vi "Exit Loop.vi"(0 "Diagram in":refnum<vi>, 1 "Loop Terminal Types":T1[](array[typedef]), 5 "Outputs":refnum<vi>[](array[refnum]), 7 "Shift Registers":refnum<vi>[](array[refnum]), 9 "Conditional Terminals":refnum<vi>[](array[refnum]), 11 "error in (no error)":errorcluster) -> (4 "Diagram out":refnum<vi>, 6 "Outputs":refnum<vi>[](array[refnum]), 8 "Shift Registers":refnum<vi>[](array[refnum]), 15 "error out":errorcluster)   [LabVIEW 2015, in "Scripting.lvlib"]
uses:
  Scripting.lvlib
  Loop Terminal Type.ctl
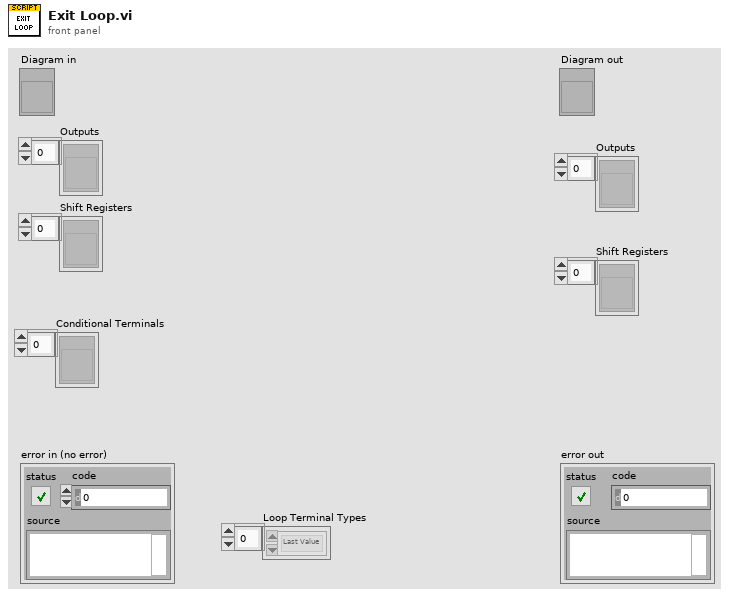
[diagram p1: front panel]
types:
  T1 = typedef "Scripting.lvlib/Loop Terminal Type.ctl" = enum16{"Last Value", "Indexing", "Concatenating"}
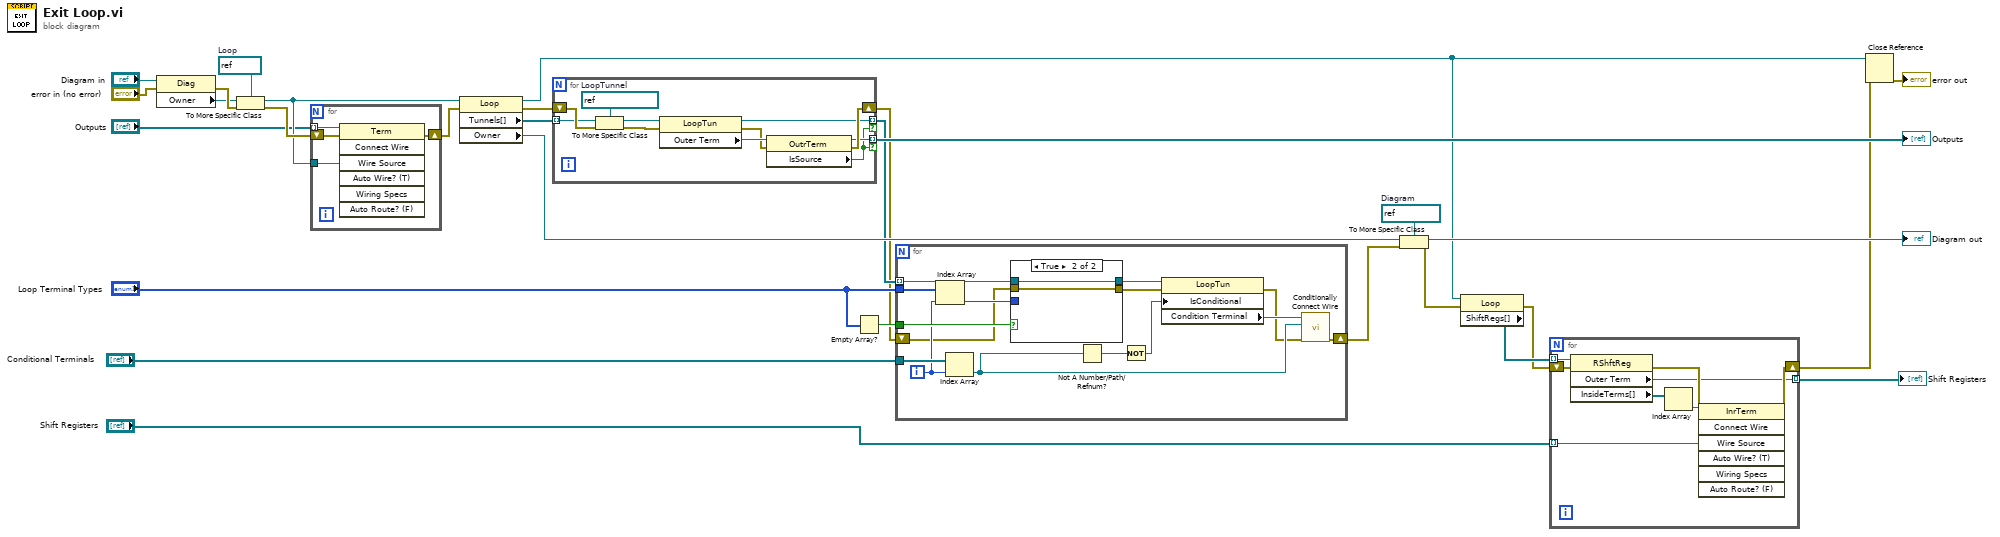
[diagram p0: block diagram]
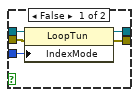
[diagram p2: hidden frame]
diagram:
  w25 = refnum<vi> refnum  # Diagram
  w27 = refnum<vi> refnum  # Loop
  n1 = property class="Diag"(reference="Diagram in", error in="error in (no error)") -> (error out=w28:errorcluster, "Owner"=w26:refnum<vi>)  [unwired: 1 out]
  n2 = To More Specific Class(target class=w27, reference=w26, error in=w28) -> (specific class reference=w24:refnum<vi>, error out=w29:errorcluster)
  n3 = for {
    tunnel: w24 -> [w32]
    shift-right: [w31] -> w23
    shift-left: w29 -> [w33]
    tunnel: "Outputs" -> [w30] mode=indexing
    n4 = invoke class="Term" method="Connect Wire"(reference=w30, error in=w33, "Wire Source"=w32) -> (error out=w31:errorcluster)  [unwired: 4 in, 6 out]
  }
  n5 = property class="Loop"(reference=w24, error in=w23) -> (reference out=w11:refnum<vi>, error out=w14:errorcluster, "Tunnels[]"=w15:refnum<vi>[], "Owner"=w16:refnum<vi>)
  n6 = for {
    tunnel: w15 -> [w38] mode=indexing
    tunnel: [w40] -> w18 mode=indexing if=w34
    shift-right: [w41] -> w3
    shift-left: w14 -> [w44]
    tunnel: [w35] -> w7 mode=indexing if=w34
    w36 = refnum<vi> refnum  # LoopTunnel
    n7 = To More Specific Class(target class=w36, reference=w38, error in=w44) -> (specific class reference=w37:refnum<vi>, error out=w39:errorcluster)
    n8 = property class="LoopTun"(reference=w37, error in=w39) -> (reference out=w35:refnum<vi>, error out=w42:errorcluster, "Outer Term"=w43:refnum<vi>)
    n9 = property class="OutrTerm"(reference=w43, error in=w42) -> (reference out=w40:refnum<vi>, error out=w41:errorcluster, "IsSource"=w34:bool)
  }
  "Outputs" <- w18
  n10 = Empty Array?(array="Loop Terminal Types") -> (empty?=w5:bool)
  n11 = for {
    tunnel: w7 -> [w59] mode=indexing
    tunnel: "Loop Terminal Types" -> [w57]
    tunnel: w5 -> [w55]
    tunnel: "Conditional Terminals" -> [w54]
    shift-right: [w46] -> w2
    shift-left: w3 -> [w52]
    i -> [w53]
    n12 = Index Array(array=w57, index=w53) -> (element=w56:T1)
    n13 = Index Array(array=w54, index=w53) -> (element=w47:refnum<vi>)
    n14 = case shown="True" w55 {
      tunnel: w59 -> [w64 w66]
      tunnel: [w63 w66] -> w58
      tunnel: w56 -> [w62 _]
      tunnel: w52 -> [w61 w65]
      tunnel: [w60 w65] -> w51
      frame False {
        n15 = property class="LoopTun"(reference=w64, error in=w61, "IndexMode"=w62) -> (reference out=w63:refnum<vi>, error out=w60:errorcluster)
      }
      frame True {
      }
    }
    n16 = Not A Number/Path/Refnum?(number/path/refnum=w47) -> (NaN/Path/Refnum?=w50:bool)
    n17 = Not(x=w50) -> (.not. x?=w49:bool)
    n18 = property class="LoopTun"(reference=w58, error in=w51, "IsConditional"=w49) -> (error out=w45:errorcluster, "Condition Terminal"=w48:refnum<vi>)  [unwired: 1 out]
    n19 = call "Conditionally Connect Wire.vi"("error in (no error)"=w45, "Wire Source"=w47, "Terminal in"=w48) -> ("error out"=w46:errorcluster)  [unwired: 7 in, 1 out]
  }
  n20 = To More Specific Class(target class=w25, reference=w16, error in=w2) -> (specific class reference=→"Diagram out":refnum<vi>, error out=w9:errorcluster)
  n21 = property class="Loop"(reference=w11, error in=w9) -> (error out=w12:errorcluster, "ShiftRegs[]"=w13:refnum<vi>[])  [unwired: 1 out]
  n22 = for {
    tunnel: w13 -> [w74] mode=indexing
    shift-right: [w69] -> w8
    shift-left: w12 -> [w71]
    tunnel: "Shift Registers" -> [w68] mode=indexing
    tunnel: [w67] -> w1 mode=indexing
    n23 = property class="RShftReg"(reference=w74, error in=w71) -> (error out=w70:errorcluster, "Outer Term"=w67:refnum<vi>, "InsideTerms[]"=w73:refnum<vi>[])  [unwired: 1 out]
    n24 = Index Array(array=w73) -> (element=w72:refnum<vi>)  [unwired: 1 in]
    n25 = invoke class="InrTerm" method="Connect Wire"(reference=w72, error in=w70, "Wire Source"=w68) -> (error out=w69:errorcluster)  [unwired: 4 in, 6 out]
  }
  "Shift Registers" <- w1
  n26 = Close Reference(reference=w11, error in (no error)=w8) -> (error out=→"error out":errorcluster)
